vi "LargeMotor.vi"() -> ()   [LabVIEW 2016, in "ENED1100-UCBA-Sensor-Motor-Testing.lvrbt"]
uses:
  ENED1100-UCBA-Sensor-Motor-Testing.lvrbt
  <vilib>/NXT/Subs/LVHSConnector.ctl
  <vilib>/NXT/LegoClasses/BrickReference/BrickReference.lvclass
  <vilib>/NXT/Block Support/NXT_OutputPort.ctl
  <vilib>/NXT/NXTIO Xnodes/NXTIONodeSubVIs/NXTMoveMotors.vi
  <vilib>/NXT/Dual Mode Library/Waits/Wait_Num.vi
  <vilib>/NXT/NXTIO Xnodes/AddressXNode/NXTIOAddress.xnode
  <vilib>/NXT/NXTIO Xnodes/NXTIOXNode/NXTIO.xnode
panel:
  out "NXT/EV3 2":T1
  in  "NXT/EV3":T1
  in  "Power/Speed 1":i8=75
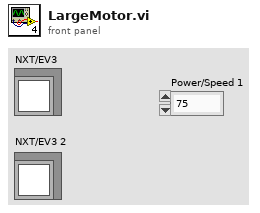
[diagram p1: front panel]
types:
  T1 = typedef "LVHSConnector.ctl" = refnum<class "BrickReference.lvclass">
  T2 = typedef "NXT_OutputPort.ctl" = u8
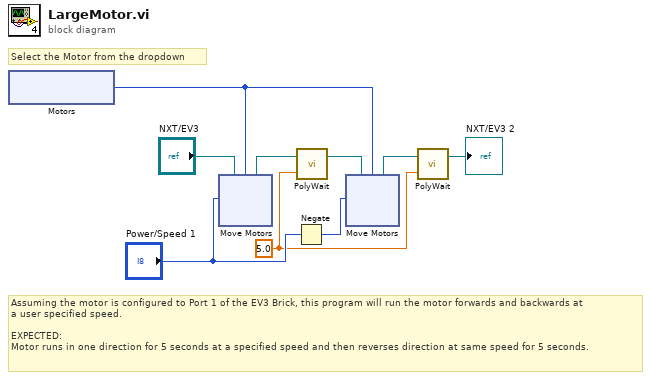
[diagram p0: block diagram]
diagram:
  w2 = sgl 5.0 ("Time (1 sec)")
  # "Assuming the motor is configured to Port 1 of the EV3 Brick, this program will run the motor forwards and backwards at\na user specified speed.\n\nEXPECTED:\nMotor runs in one direction for 5 seconds at a specified speed and then reverses direction at same speed for 5 seconds."
  # "Select the Motor from the dropdown"
  n1 = xnode "Motors"() -> ("Motor"=w4:T2)
  n2 = xnode "Move Motors"("Power/Speed 1"="Power/Speed 1", "Motors"=w4, "NXT/EV3"="NXT/EV3") -> ("NXT/EV3"=w9:T1)
  n3 = Negate(x="Power/Speed 1") -> (-x=w5:i8)
  n4 = call-poly <vilib>:"PolyWait.vi"("Time (1 sec)"=w2, "NXT/EV3"=w9) -> ("NXT/EV3"=w8:T1)  [unwired: 2 in]
  n5 = xnode "Move Motors"("Power/Speed 1"=w5, "Motors"=w4, "NXT/EV3"=w8) -> ("NXT/EV3"=w3:T1)
  n6 = call-poly <vilib>:"PolyWait.vi"("Time (1 sec)"=w2, "NXT/EV3"=w3) -> ("NXT/EV3"=→"NXT/EV3 2":T1)  [unwired: 2 in]
